vi "旁路系统.vi"() -> ()   [LabVIEW 2016, in "质控单元V4.lvlib"]
uses:
  <vilib>/Utility/config.llb/NI_LVConfig.lvlib
panel:
  in  "选择参数":bool
  in  "参数设置":T1={"沉淀时间 1"=30, "浊度阀值 1"=200.0, "浊度阀值 2"=500.0, "沉淀时间 2"=40} {"沉淀时间 2" format="%d min"; "浊度阀值 2" format="%.2f NTU"; "浊度阀值 1" format="%.2f NTU"; "沉淀时间 1" format="%d min"}
  in  "启动设置":u16(ring) items=["手动", "自动"]
  out "当前浊度":dbl format="%.2f NTU"
  out "工作状态":bool
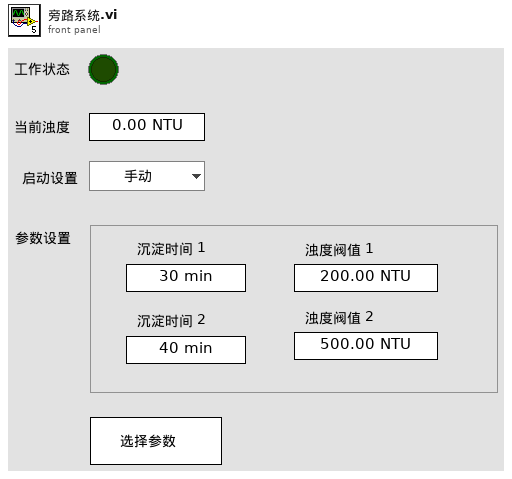
[diagram p1: front panel]
types:
  T1 = cluster{"沉淀时间 1":i32, "浊度阀值 1":dbl, "浊度阀值 2":dbl, "沉淀时间 2":i32}
  T2 = typedef "NI_LVConfig.lvlib/Config Data RefNum.ctl" = refnum<k1>
  T3 = cluster{"水样数据时间":timestamp, "水温":dbl, "pH":dbl, "DO":dbl, "DOper":dbl, "电导率":dbl, "ORP":dbl, "浊度":dbl, "叶绿素a":dbl, "藻密度":dbl, "COD":dbl, "DO2":dbl, "DO2per":dbl, "氯化物":dbl, "氨氮":dbl, "水中油":dbl}
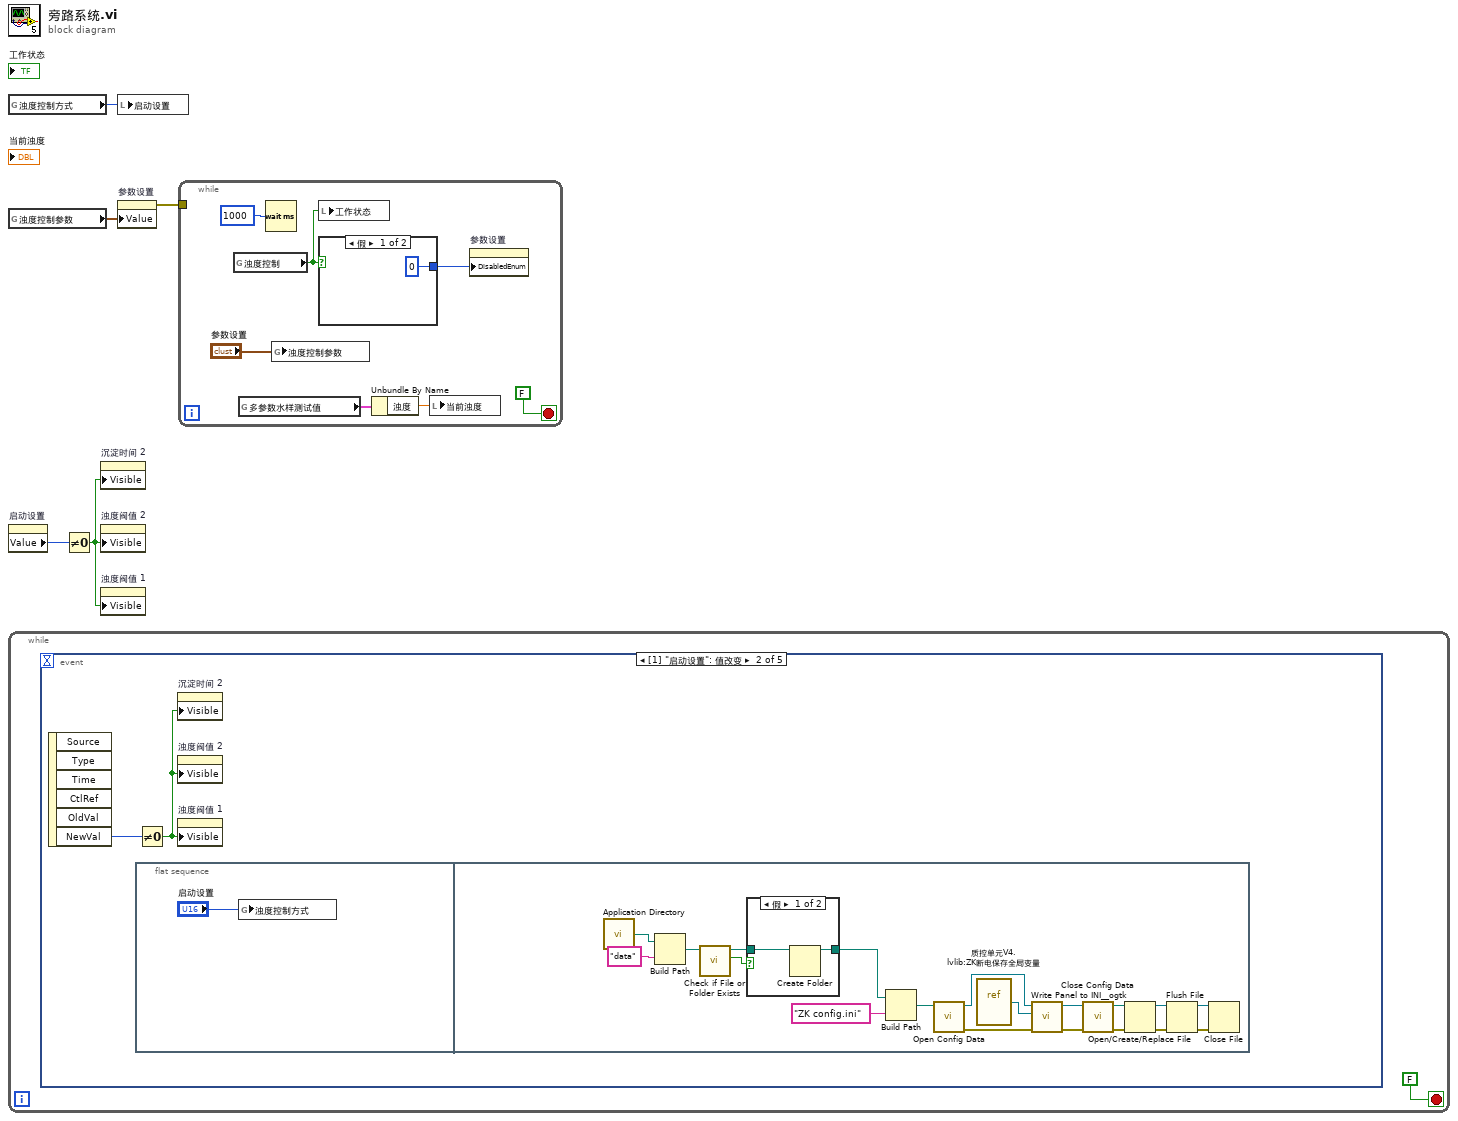
[diagram p0: block diagram]
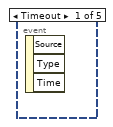
[diagram p2: hidden frame]
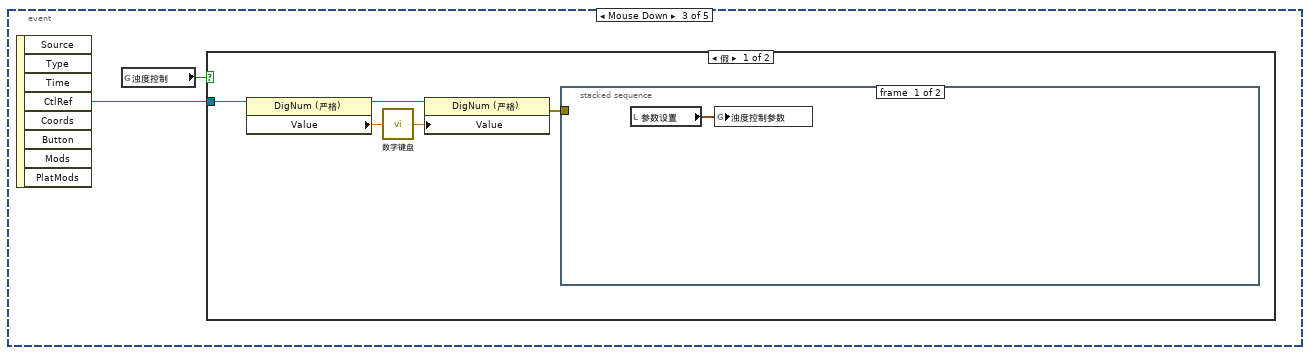
[diagram p4: hidden frame]
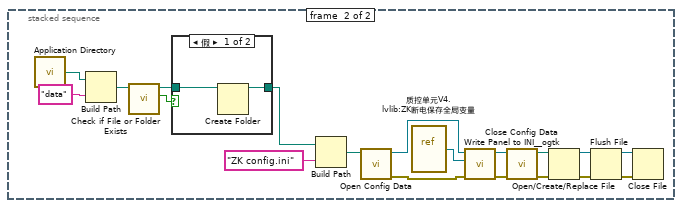
[diagram p5: hidden frame]
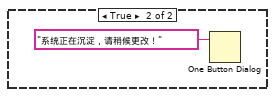
[diagram p7: hidden frame]
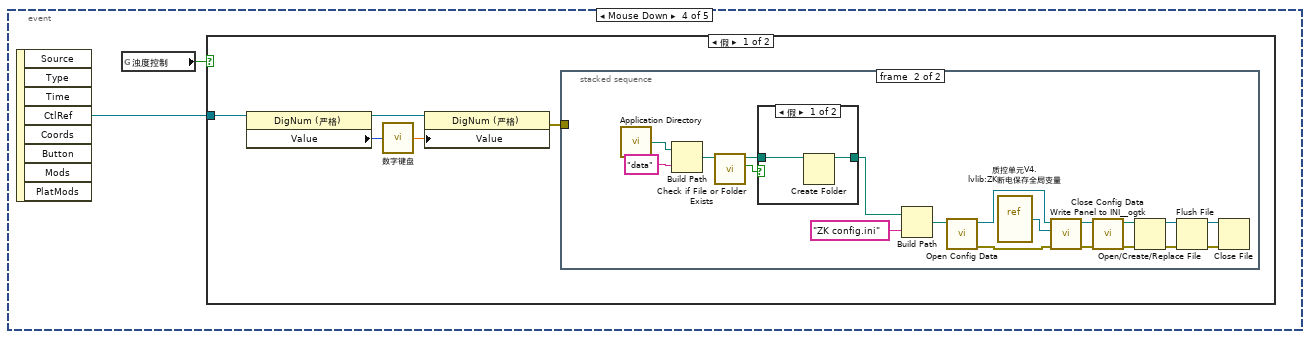
[diagram p8: hidden frame]
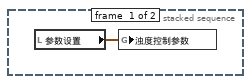
[diagram p9: hidden frame]
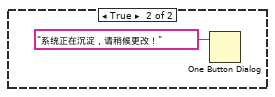
[diagram p11: hidden frame]
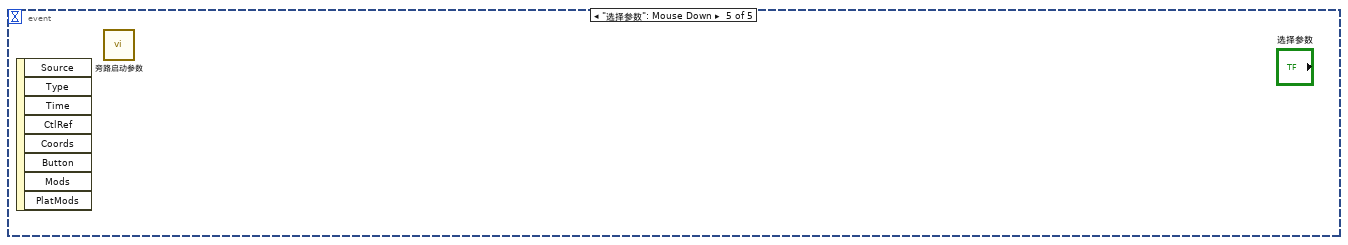
[diagram p12: hidden frame]
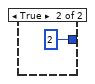
[diagram p13: hidden frame]
diagram:
  n1 = global read "ZK断电保存全局变量.vi" "浊度控制方式"() -> (w1:u16)
  n2 = global read "ZK断电保存全局变量.vi" "浊度控制参数"() -> (w5:T1)
  n3 = property on="启动设置" class="Ring (严格)"() -> ("Value"=w2:u16)  [unwired: 2 in, 2 out]
  n4 = while {
    stop <- FALSE stop-if-true
    n5 = event shown="[1] \"启动设置\": 值改变" {
      selector: _ -> [_ _ _ _ _]
      dyn-events: _ -> [_ _ _ _ _]
      timeout: _ -> [_ _ _ _ _]
      event Timeout {
        n6 = event-data() -> ()  [unwired: 1 in, 3 out]
      }
      event "启动设置": Value Change {
        n7 = event-data() -> ("NewVal"=w8:u16)  [unwired: 1 in, 5 out]
        n8 = flat-sequence {
          frame #0 {
            n9 = global write "ZK断电保存全局变量.vi" "浊度控制方式"("启动设置") -> ()
          }
          frame #1 {
            n10 = call <vilib>:"Application Directory.vi"() -> ("Application Directory"=w11:path)
            n11 = Build Path(base path=w11, name or relative path="data" ("名称或相对路径")) -> (appended path=w13:path)
            n12 = call <vilib>:"Check if File or Folder Exists.vi"("path"=w13) -> ("file or folder exists?"=w14:bool, "dup path"=w15:path)  [unwired: 8 in, 1 out]
            n13 = case shown="假" w14 {
              tunnel: w15 -> [w30 w31]
              tunnel: [w29 w31] -> w16
              frame False {
                n14 = Create Folder(path (use dialog)=w30) -> (created path=w29:path)  [unwired: 2 in, 2 out]
              }
              frame True {
              }
            }
            n15 = Build Path(base path=w16, name or relative path="ZK config.ini" ("名称或相对路径")) -> (appended path=w10:path)
            n16 = call <vilib>:"Open Config Data.vi"("configuration file path"=w10) -> ("error out"=w21:errorcluster, "refnum"=w19:T2)  [unwired: 8 in, 1 out]
            n17 = vi-ref "质控单元V4.lvlib:ZK断电保存全局变量.vi"() -> (w18:refnum<vi>)
            n18 = call <userlib>:"Write Panel to INI__ogtk.vi"("error in (no error)"=w21, "VI ref"=w18, "refnum"=w19) -> ("error out"=w22:errorcluster, "refnum out"=w20:T2)  [unwired: 7 in]
            n19 = call <vilib>:"Close Config Data.vi"("error in (no error)"=w22, "refnum"=w20) -> ("error out"=w27:errorcluster, "file path"=w28:path)  [unwired: 8 in]
            n20 = Open/Create/Replace File(file path (use dialog)=w28, error in=w27) -> (refnum out=w24:refnum<file>, error out=w23:errorcluster)  [unwired: 4 in, 1 out]
            n21 = Flush File(refnum=w24, error in=w23) -> (refnum out=w25:refnum<file>, error out=w26:errorcluster)
            n22 = Close File(refnum=w25, error in=w26) -> ()  [unwired: 2 out]
          }
        }
        n23 = Not Equal To 0?(x=w8) -> (x != 0?=w7:bool)
        n24 = property on="沉淀时间 2" class="DigNum (严格)"("Visible"=w7) -> ()  [unwired: 2 in, 2 out]
        n25 = property on="浊度阀值 2" class="DigNum (严格)"("Visible"=w7) -> ()  [unwired: 2 in, 2 out]
        n26 = property on="浊度阀值 1" class="DigNum (严格)"("Visible"=w7) -> ()  [unwired: 2 in, 2 out]
      }
      event "参数设置.浊度阀值 1", "参数设置.浊度阀值 2": Mouse Down {
        n27 = event-data() -> ("CtlRef"=w33:refnum<vi>)  [unwired: 1 in, 7 out]
        n28 = global read "ZK断电保存全局变量.vi" "浊度控制"() -> (w32:bool)
        n29 = case shown="假" w32 {
          tunnel: w33 -> [w35 _]
          frame False {
            n30 = property class="DigNum (严格)"(reference=w35) -> (reference out=w37:refnum<vi>, "Value"=w38:dbl)  [unwired: 1 in, 1 out]
            n31 = call "数字键盘.vi"("OldNumber"=w38) -> ("NewNumber"=w36:sgl)
            n32 = property class="DigNum (严格)"(reference=w37, "Value"=w36) -> (error out=w34:errorcluster)  [unwired: 1 in, 1 out]
            n33 = stacked-sequence {
              tunnel: w34 -> [_ _]
              frame #0 {
                n34 = local read "参数设置"() -> (w39:T1)
                n35 = global write "ZK断电保存全局变量.vi" "浊度控制参数"(w39) -> ()
              }
              frame #1 {
                n36 = call <vilib>:"Application Directory.vi"() -> ("Application Directory"=w41:path)
                n37 = Build Path(base path=w41, name or relative path="data" ("名称或相对路径")) -> (appended path=w43:path)
                n38 = call <vilib>:"Check if File or Folder Exists.vi"("path"=w43) -> ("file or folder exists?"=w44:bool, "dup path"=w45:path)  [unwired: 8 in, 1 out]
                n39 = case shown="假" w44 {
                  tunnel: w45 -> [w60 w61]
                  tunnel: [w59 w61] -> w46
                  frame False {
                    n40 = Create Folder(path (use dialog)=w60) -> (created path=w59:path)  [unwired: 2 in, 2 out]
                  }
                  frame True {
                  }
                }
                n41 = Build Path(base path=w46, name or relative path="ZK config.ini" ("名称或相对路径")) -> (appended path=w40:path)
                n42 = call <vilib>:"Open Config Data.vi"("configuration file path"=w40) -> ("error out"=w51:errorcluster, "refnum"=w49:T2)  [unwired: 8 in, 1 out]
                n43 = vi-ref "质控单元V4.lvlib:ZK断电保存全局变量.vi"() -> (w48:refnum<vi>)
                n44 = call <userlib>:"Write Panel to INI__ogtk.vi"("error in (no error)"=w51, "VI ref"=w48, "refnum"=w49) -> ("error out"=w52:errorcluster, "refnum out"=w50:T2)  [unwired: 7 in]
                n45 = call <vilib>:"Close Config Data.vi"("error in (no error)"=w52, "refnum"=w50) -> ("error out"=w57:errorcluster, "file path"=w58:path)  [unwired: 8 in]
                n46 = Open/Create/Replace File(file path (use dialog)=w58, error in=w57) -> (refnum out=w54:refnum<file>, error out=w53:errorcluster)  [unwired: 4 in, 1 out]
                n47 = Flush File(refnum=w54, error in=w53) -> (refnum out=w55:refnum<file>, error out=w56:errorcluster)
                n48 = Close File(refnum=w55, error in=w56) -> ()  [unwired: 2 out]
              }
            }
          }
          frame True {
            n49 = One Button Dialog(message="系统正在沉淀，请稍候更改！" ("消息")) -> ()  [unwired: 1 in, 1 out]
          }
        }
      }
      event "参数设置.沉淀时间 1", "参数设置.沉淀时间 2": Mouse Down {
        n50 = event-data() -> ("CtlRef"=w64:refnum<vi>)  [unwired: 1 in, 7 out]
        n51 = global read "ZK断电保存全局变量.vi" "浊度控制"() -> (w63:bool)
        n52 = case shown="假" w63 {
          tunnel: w64 -> [w66 _]
          frame False {
            n53 = property class="DigNum (严格)"(reference=w66) -> (reference out=w68:refnum<vi>, "Value"=w69:i32)  [unwired: 1 in, 1 out]
            n54 = call "数字键盘.vi"("OldNumber"=w69) -> ("NewNumber"=w67:sgl)
            n55 = property class="DigNum (严格)"(reference=w68, "Value"=w67) -> (error out=w65:errorcluster)  [unwired: 1 in, 1 out]
            n56 = stacked-sequence {
              tunnel: w65 -> [_ _]
              frame #0 {
                n57 = local read "参数设置"() -> (w70:T1)
                n58 = global write "ZK断电保存全局变量.vi" "浊度控制参数"(w70) -> ()
              }
              frame #1 {
                n59 = call <vilib>:"Application Directory.vi"() -> ("Application Directory"=w72:path)
                n60 = Build Path(base path=w72, name or relative path="data" ("名称或相对路径")) -> (appended path=w74:path)
                n61 = call <vilib>:"Check if File or Folder Exists.vi"("path"=w74) -> ("file or folder exists?"=w75:bool, "dup path"=w76:path)  [unwired: 8 in, 1 out]
                n62 = case shown="假" w75 {
                  tunnel: w76 -> [w91 w92]
                  tunnel: [w90 w92] -> w77
                  frame False {
                    n63 = Create Folder(path (use dialog)=w91) -> (created path=w90:path)  [unwired: 2 in, 2 out]
                  }
                  frame True {
                  }
                }
                n64 = Build Path(base path=w77, name or relative path="ZK config.ini" ("名称或相对路径")) -> (appended path=w71:path)
                n65 = call <vilib>:"Open Config Data.vi"("configuration file path"=w71) -> ("error out"=w82:errorcluster, "refnum"=w80:T2)  [unwired: 8 in, 1 out]
                n66 = vi-ref "质控单元V4.lvlib:ZK断电保存全局变量.vi"() -> (w79:refnum<vi>)
                n67 = call <userlib>:"Write Panel to INI__ogtk.vi"("error in (no error)"=w82, "VI ref"=w79, "refnum"=w80) -> ("error out"=w83:errorcluster, "refnum out"=w81:T2)  [unwired: 7 in]
                n68 = call <vilib>:"Close Config Data.vi"("error in (no error)"=w83, "refnum"=w81) -> ("error out"=w88:errorcluster, "file path"=w89:path)  [unwired: 8 in]
                n69 = Open/Create/Replace File(file path (use dialog)=w89, error in=w88) -> (refnum out=w85:refnum<file>, error out=w84:errorcluster)  [unwired: 4 in, 1 out]
                n70 = Flush File(refnum=w85, error in=w84) -> (refnum out=w86:refnum<file>, error out=w87:errorcluster)
                n71 = Close File(refnum=w86, error in=w87) -> ()  [unwired: 2 out]
              }
            }
          }
          frame True {
            n72 = One Button Dialog(message="系统正在沉淀，请稍候更改！" ("消息")) -> ()  [unwired: 1 in, 1 out]
          }
        }
      }
      event "选择参数": Mouse Down {
        n73 = event-data() -> ()  [unwired: 1 in, 8 out]
        n74 = call "旁路启动参数.vi"() -> ()  [unwired: 12 in]
      }
    }
  }
  n75 = Not Equal To 0?(x=w2) -> (x != 0?=w3:bool)
  n76 = property on="沉淀时间 2" class="DigNum (严格)"("Visible"=w3) -> ()  [unwired: 2 in, 2 out]
  n77 = property on="浊度阀值 2" class="DigNum (严格)"("Visible"=w3) -> ()  [unwired: 2 in, 2 out]
  n78 = property on="浊度阀值 1" class="DigNum (严格)"("Visible"=w3) -> ()  [unwired: 2 in, 2 out]
  n79 = local write "启动设置"(w1) -> ()
  n80 = property on="参数设置" class="Clust (严格)"("Value"=w5) -> (error out=w4:errorcluster)  [unwired: 2 in, 1 out]
  n81 = while {
    tunnel: w4 -> [_]
    stop <- FALSE stop-if-true
    n82 = global read "ZK断电保存全局变量.vi" "浊度控制"() -> (w95:bool)
    n83 = global read "多参数全局变量.vi" "多参数水样测试值"() -> (w97:T3)
    n84 = Wait (ms)(milliseconds to wait=u32 1000 ("等待时间（毫秒）")) -> ()  [unwired: 1 out]
    n85 = global write "ZK断电保存全局变量.vi" "浊度控制参数"("参数设置") -> ()
    n86 = local write "工作状态"(w95) -> ()
    n87 = case shown="假" w95 {
      tunnel: [0 2] -> w94
      frame False {
      }
      frame True {
      }
    }
    n88 = Unbundle By Name(w97) -> ("浊度"=w98:dbl)
    n89 = local write "当前浊度"(w98) -> ()
    n90 = property on="参数设置" class="Clust (严格)"("DisabledEnum"=w94) -> ()  [unwired: 2 in, 2 out]
  }
